vi "Init Root Log.vi"(8 "error in (no error)":errorcluster, 11 "CoolAppProcess in":refnum<class "CoolAppProcess.lvclass">) -> (0 "error out":errorcluster, 3 "CoolAppProcess out":refnum<class "CoolAppProcess.lvclass">)   [LabVIEW 2020, in "LAF2024Q2.lvlib" / "CoolAppProcess.lvclass"]
uses:
  CoolAppProcess.lvclass
  CoolAppProcess.lvclass/CoolAppProcess.ctl
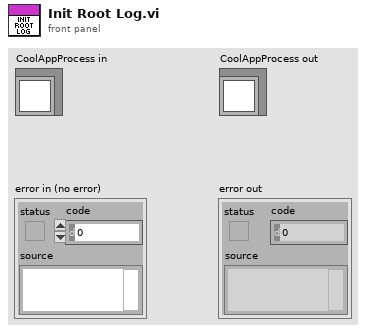
[diagram p1: front panel]
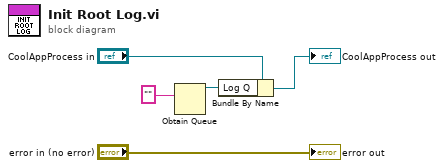
[diagram p0: block diagram]
diagram:
  n1 = Obtain Queue(element data type="") -> (queue out=w3:refnum<queue>)  [unwired: 4 in, 2 out]
  n2 = Bundle By Name(cluster="CoolAppProcess in", "Log Q"=w3) -> (→"CoolAppProcess out":refnum<class "CoolAppProcess.lvclass">)
  "error out" <- "error in (no error)"
